vi "Float to Little Endian Byte Array.vi"(11 "Float In":sgl) -> (3 "LE Byte Array":u8[](array[numeric]))   [LabVIEW 2014]
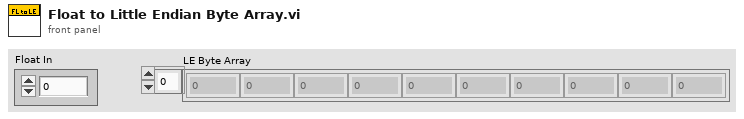
[diagram p1: front panel]
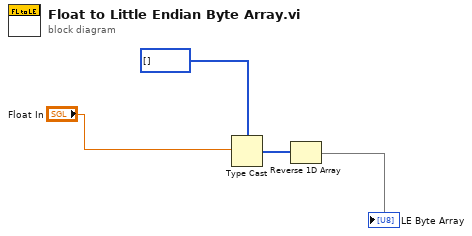
[diagram p0: block diagram]
diagram:
  n1 = Type Cast(type=u8[] [], x="Float In") -> (*(type *) &x=w2:u8[])
  n2 = Reverse 1D Array(array=w2) -> (reversed array=→"LE Byte Array":u8[])
